vi "PH_gentec_P-Link.get current Measurement.vi"(0 "i ref in":refnum<vi>, 2 "VISA resource in":refnum<visa-resource-name>, 5 "error in":errorcluster) -> (11 "Timeout":bool, 13 "Data read":string[](array[string]), 14 "i ref out":refnum<vi>, 16 "VISA resource out":refnum<visa-resource-name>, 17 "Error":bool, 19 "error out":errorcluster)   [LabVIEW 2014, in "PH_gentec_P-Link.lvlib"]
doc: "This VI writes wanted Settings to the Device and checks the result."
uses:
  PH_gentec_P-Link.lvlib
  PH_Basics/PH_Powermeter_BaseClass/PH_Powermeter_BaseClass.lvlib
  instr.lib/Gentec-P-Link/gentec-P-Link - Driver.lvlib
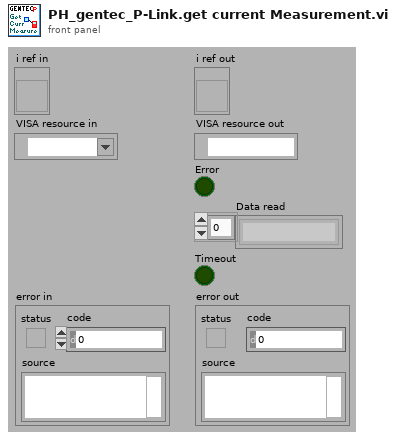
[diagram p1: front panel]
types:
  T1 = typedef "PH_gentec_P-Link.lvlib/PH_gentec_P-Link.i attribute.ctl" = cluster{"GUI References":cluster{"Wanted Head Settings":refnum<vi>, "Current Head Settings":refnum<vi>, "Set Auto Range":refnum<vi>, "Trigger Polarity":refnum<vi>, "Trigger Source":refnum<vi>, "Waveform Averages":refnum<vi>, "Continuous":refnum<vi>, "get one Value":refnum<vi>}, "Wanted Head Settings":T2, "Current Head Settings":T2}
  T2 = typedef "PH_gentec_P-Link.lvlib/PH_gentec_P-Link.Head Settings.ctl" = cluster{"Measurement Mode":T3, "Enable Anticipation":bool, "Set Auto Range":bool, "Block Signal":bool, "Set Head Attenuator":bool, "Enable SSE":bool, "Trigger Polarity":T4, "Trigger Source":T5, "Waveform Averages":T6, "Set Zero":i32, "Current":i32, "Start Data Flow":bool}
  T3 = typedef "gentec-M-Link - Driver.lvlib/gentec-M-Link.Measurement Mode.ctl" = u16
  T4 = typedef "gentec-M-Link - Driver.lvlib/gentec-M-Link.Trigger Polarity.ctl" = u16
  T5 = typedef "gentec-M-Link - Driver.lvlib/gentec-M-Link.Trigger Source.ctl" = u16
  T6 = typedef "gentec-M-Link - Driver.lvlib/gentec-M-Link.Waveform Averages.ctl" = u16
  T7 = typedef "PH_Powermeter_BaseClass.lvlib/PH_Powermeter_BaseClass.i attribute.ctl" = cluster{"GUI References":T8, "Connection":T9, "Head Attributes":T11, "VISA resource":refnum<visa-resource-name>, "Energy":T12, "Service ID Energy":i32, "Wanted Settings":T13, "Current Settings":T13}
  T8 = typedef "PH_Powermeter_BaseClass.lvlib/PH_Powermeter_BaseClass.GUI Refs.ctl" = cluster{"Head Attributes":refnum<vi>, "Energy":refnum<vi>, "Connection":refnum<vi>, "VISA Resource":refnum<vi>, "Scaling Factor":refnum<vi>, "Range":refnum<vi>, "Wavelength":refnum<vi>, "Trigger Level":refnum<vi>, "Wanted Settings":refnum<vi>, "Current Settings":refnum<vi>}
  T9 = typedef "PH_Powermeter_BaseClass.lvlib/PH_Powermeter_BaseClass.Connection.ctl" = cluster{"failed checks":i8, "Timeout":bool, "Data read":string, "Failure":bool, "Error":bool, "State":T10}
  T10 = typedef "PH_Powermeter_BaseClass.lvlib/PH_Powermeter_BaseClass.State.ctl" = enum32{"off", "operating", "opened", "checked", "connected", "Sets to change", "running"}
  T11 = typedef "PH_Powermeter_BaseClass.lvlib/PH_Powermeter_BaseClass.Head Attributes.ctl" = cluster{"Instrument Type":string, "Head Version":string, "Head Name":string, "Serial Number":string, "Firmware":string, "Sensor Type":string, "MinimumRange":u32, "Maximum Range":u32, "Min Wavelength":i32, "Max Wavelength":i32}
  T12 = typedef "PH_Powermeter_BaseClass.lvlib/PH_Powermeter_BaseClass.Energy.ctl" = cluster{"current Value":dbl, "unscaled":dbl, "Scaling Factor":dbl}
  T13 = typedef "PH_Powermeter_BaseClass.lvlib/PH_gentec_BaseClass.Head Settings.ctl" = cluster{"Trigger Level":dbl, "Wavelength":u32, "Range":u32}
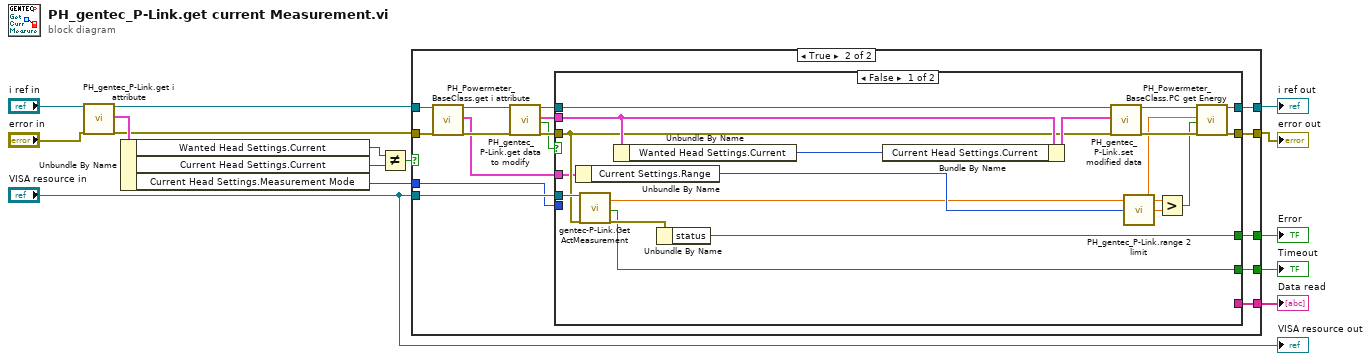
[diagram p0: block diagram]
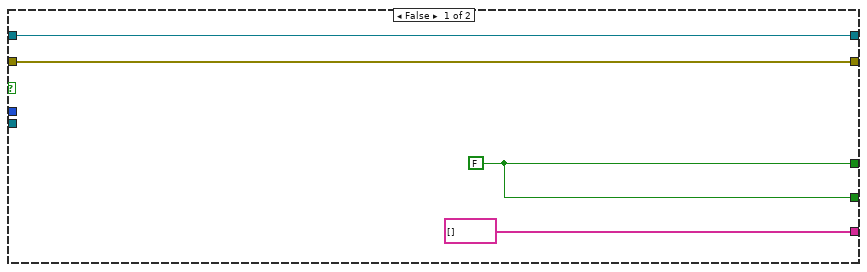
[diagram p2: hidden frame]
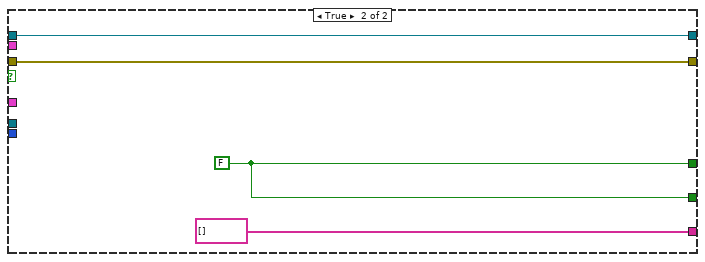
[diagram p3: hidden frame]
diagram:
  n1 = call "PH_gentec_P-Link.get i attribute.vi"("i ref in"="i ref in", "error in (no error)"="error in") -> ("i ref out"=w9:refnum<vi>, "i attribute"=w12:T1, "error out"=w11:errorcluster)  [unwired: 15 in]
  n2 = Unbundle By Name(w12) -> ("Wanted Head Settings.Current"=w13:i32, "Current Head Settings.Current"=w2:i32, "Current Head Settings.Measurement Mode"=w1:T3)
  n3 = Not Equal?(x=w13, y=w2) -> (x != y?=w3:bool)
  n4 = case shown="True" w3 {
    tunnel: [w16 w35] -> w15
    tunnel: [w17 w34] -> w14
    tunnel: w11 -> [w16 w29]
    tunnel: w9 -> [w17 w23]
    tunnel: "VISA resource in" -> [_ w28]
    tunnel: [w19 w27] -> w6
    tunnel: [w19 w26] -> w5
    tunnel: [string[] [] w20] -> w4
    tunnel: w1 -> [_ w25]
    frame False {
      w19 = FALSE
    }
    frame True {
      n5 = call "PH_Powermeter_BaseClass.get i attribute.vi"("i ref in"=w23, "error in (no error)"=w29) -> ("i ref out"=w22:refnum<vi>, "i attribute"=w21:T7, "error out"=w24:errorcluster)  [unwired: 15 in]
      n6 = call "PH_gentec_P-Link.get data to modify.vi"("i ref in"=w22, "error in (no error)"=w24) -> ("i ref out"=w32:refnum<vi>, "i attribute"=w31:T1, "timed out"=w30:bool, "error out"=w33:errorcluster)  [unwired: 14 in]
      n7 = case shown="False" w30 {
        tunnel: w28 -> [w53 _]
        tunnel: [w44 w57] -> w34
        tunnel: [w46 w56] -> w35
        tunnel: w33 -> [w40 w56]
        tunnel: w32 -> [w41 w57]
        tunnel: w31 -> [w48 _]
        tunnel: [w50 w55] -> w27
        tunnel: [w36 w55] -> w26
        tunnel: w25 -> [_ _]
        tunnel: w21 -> [w39 _]
        tunnel: [_ string[] []] -> w20
        frame False {
          n8 = Unbundle By Name(w39) -> ("Current Settings.Range"=w38:u32)
          n9 = call "gentec-P-Link.Get ActMeasurement.vi"("VISA resource name"=w53, "error in (no error)"=w40) -> ("Measurement"=w37:dbl, "TimeOut?"=w36:bool, "error out"=w49:errorcluster)  [unwired: 13 in, 2 out]
          n10 = Unbundle By Name(w48) -> ("Wanted Head Settings.Current"=w47:i32)
          n11 = Unbundle By Name(w49) -> ("status"=w50:bool)
          n12 = Bundle By Name(cluster=w48, "Current Head Settings.Current"=w47) -> (w51:T1)
          n13 = call "PH_gentec_P-Link.set modified data.vi"("i ref in"=w41, "i attribute"=w51, "error in (no error)"=w40) -> ("i ref out"=w45:refnum<vi>, "error out"=w52:errorcluster)  [unwired: 15 in]
          n14 = call "PH_gentec_P-Link.range 2 limit.vi"("Range"=w38) -> ("limit"=w43:dbl)
          n15 = Greater?(x=w37, y=w43) -> (0:w42:bool)
          n16 = call "PH_Powermeter_BaseClass.PC get Energy.vi"("i ref in"=w45, "unscaled Energy [J]"=w37, "Out of range?"=w42, "error in"=w52) -> ("i ref out"=w44:refnum<vi>, "error out"=w46:errorcluster)  [unwired: 14 in]
        }
        frame True {
          w55 = FALSE
        }
      }
    }
  }
  "error out" <- w15
  "i ref out" <- w14
  "Error" <- w6
  "Timeout" <- w5
  "Data read" <- w4
  "VISA resource out" <- "VISA resource in"
